vi "DataLog Sort Tag Info List.vi"(7 "tag list in":T1[](array[typedef]) {"logging parameters" format="%.2e"; "precision" items=["0", "1", "2", "3", "4", "5", "6", "7", "8", "9", "10", "11", "12", "13", "14", "15", "16", "17"]; "limit delay" format="%.2e"; "deadband" format="%.2e"}) -> (8 "tag list out":T1[](array[typedef]) {"logging parameters" format="%.2e"; "precision" items=["0", "1", "2", "3", "4", "5", "6", "7", "8", "9", "10", "11", "12", "13", "14", "15", "16", "17"]; "limit delay" format="%.2e"; "deadband" format="%.2e"})   [LabVIEW 2012]
doc: "Searches for a tag in the provided tag info list and returns the index in the list as well as the tag's info. When the data logging is active, the tag hash should be used so as to perform the index lookup much more efficiently."
uses:
  typedefs/clusters/t_DataLog Tag Config.ctl
  typedefs/t_DataLog Temporal Types.ctl
  typedefs/t_DataLog Value Types.ctl
  typedefs/t_DataLog Numerical Format.ctl
  typedefs/t_DataLog Logging Algorithms.ctl
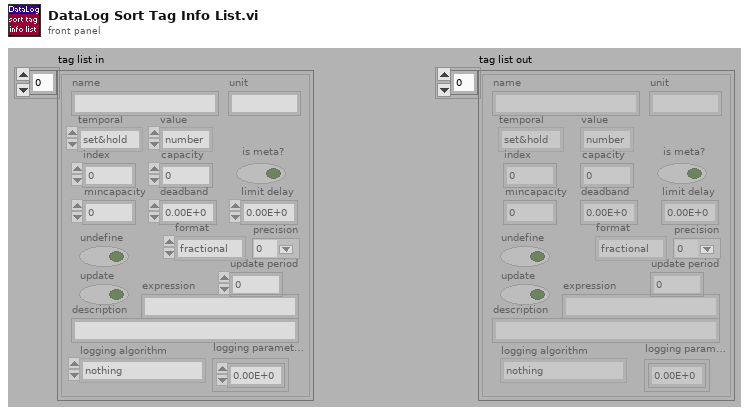
[diagram p1: front panel]
types:
  T1 = typedef "t_DataLog Tag Config.ctl" = cluster{"name":string, "unit":string, "temporal":T2, "value":T3, "index":i32, "capacity":i32, "is meta?":bool, "mincapacity":i32, "deadband":dbl, "limit delay":dbl, "format":T4, "precision":u8, "undefine":bool, "update":bool, "update period":u16, "expression":string, "description":string, "logging algorithm":T5, "logging parameters":dbl[]}
  T2 = typedef "t_DataLog Temporal Types.ctl" = enum16{"set&hold", "sample", "event"}
  T3 = typedef "t_DataLog Value Types.ctl" = enum16{"number", "string"}
  T4 = typedef "t_DataLog Numerical Format.ctl" = enum8{"fractional", "exponential", "engineering"}
  T5 = typedef "t_DataLog Logging Algorithms.ctl" = enum16{"nothing", "changes", "everything", "every Nth", "time threshold", "value threshold + prior", "t or v threshold", "t or v threshold + prior"}
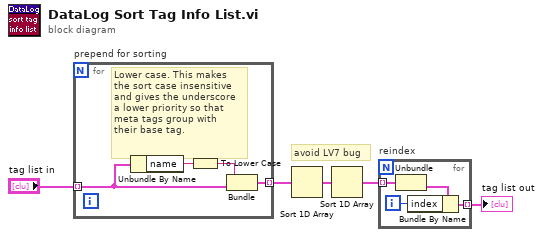
[diagram p0: block diagram]
diagram:
  # "avoid LV7 bug"
  n1 = for "prepend for sorting" {
    tunnel: "tag list in" -> [w8] mode=indexing
    tunnel: [w7] -> w4 mode=indexing
    # "Lower case. This makes\nthe sort case insensitive\nand gives the underscore\na lower priority so that\nmeta tags group with\ntheir base tag."
    n2 = Unbundle By Name(w8) -> ("name"=w9:string)
    n3 = To Lower Case(string=w9) -> (all lower case string=w6:string)
    n4 = Bundle(w6, w8) -> (w7:cluster{string, T1})  [unwired: 1 in]
  }
  n5 = Sort 1D Array(array=w4) -> (sorted array=w2:cluster{string, T1}[])
  n6 = Sort 1D Array(array=w2) -> (sorted array=w1:cluster{string, T1}[])
  n7 = for "reindex" {
    tunnel: w1 -> [w12] mode=indexing
    tunnel: [w13] -> w3 mode=indexing
    i -> [w11]
    n8 = Unbundle(w12) -> (w10:T1)  [unwired: 1 out]
    n9 = Bundle By Name(cluster=w10, "index"=w11) -> (w13:T1)
  }
  "tag list out" <- w3
